vi "LINC Register LabVIEW File.vi"(4 "alternate packet names (empty)":string[](array[string]), 5 "ID":i32=-1, 6 "control names (empty)":string[](array[string]), 7 "mode (exclude)":enum16{"exclude", "include"}(ring), 8 "error in (no error)":errorcluster, 9 "type (CMD)":enum16{"CMD", "TLM", "CMD_HDR", "TLM_HDR"}(ring), 10 "prototype path":path, 11 "LINC session":refnum<class "LINC.lvclass">) -> (0 "error out":errorcluster, 3 "dup LINC session":refnum<class "LINC.lvclass">)   [LabVIEW 2018, in "STEPkgDriver_LINC.lvlib" / "LINC.lvclass"]
uses:
  LINC.lvclass
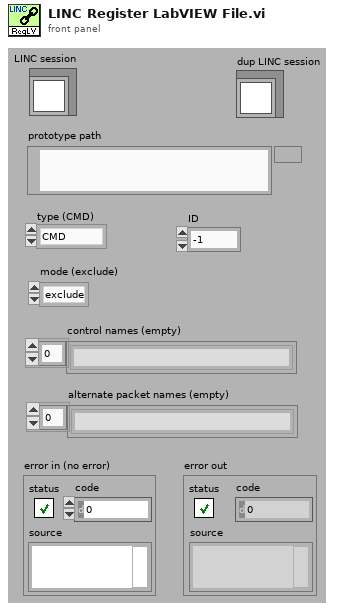
[diagram p1: front panel]
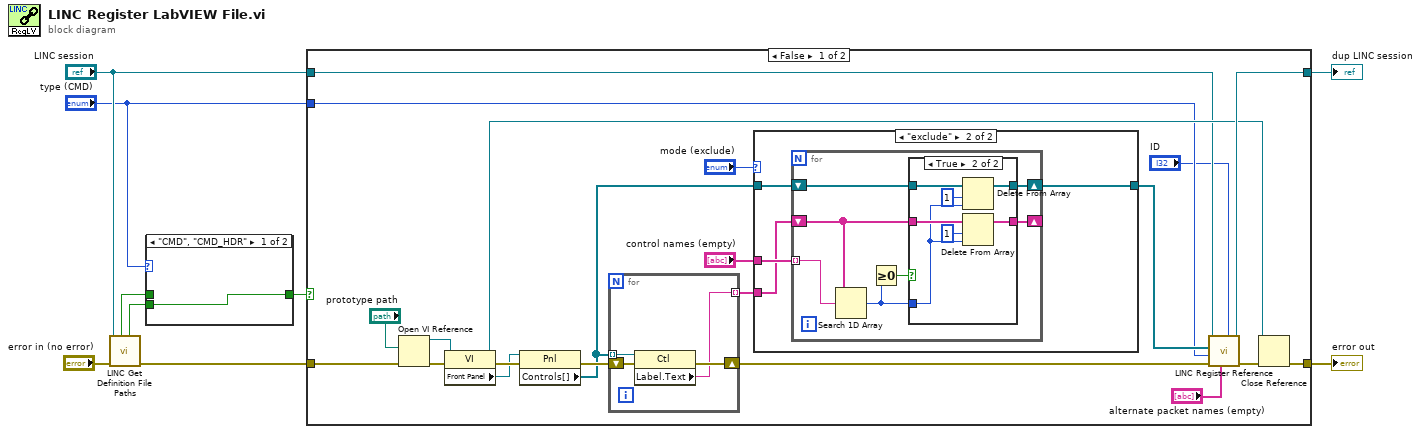
[diagram p0: block diagram]
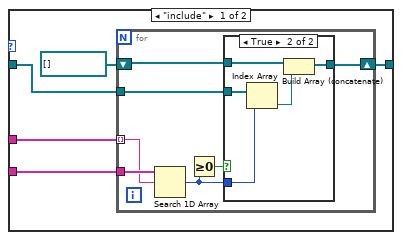
[diagram p2: hidden frame]
diagram:
  n1 = call "LINC Get Definition File Paths.vi"("error in (no error)"="error in (no error)", "LINC session"="LINC session") -> ("error out"=w5:errorcluster, "CMD definition exists"=w6:bool, "TLM definition exists"=w7:bool)  [unwired: 4 in, 3 out]
  n2 = case shown="\"CMD\", \"CMD_HDR\"" "type (CMD)" {
    tunnel: w7 -> [_ w11]
    tunnel: w6 -> [w10 _]
    tunnel: [w10 w11] -> w2
    frame "CMD", "CMD_HDR" {
    }
    frame "TLM", "TLM_HDR" {
    }
  }
  n3 = case shown="False" w2 {
    tunnel: [w20 w76] -> w9
    tunnel: [w19 w75] -> w8
    tunnel: w5 -> [w15 w76]
    tunnel: "LINC session" -> [w14 w75]
    tunnel: "type (CMD)" -> [w13 _]
    frame False {
      n4 = Open VI Reference(vi path="prototype path", error in (no error)=w15) -> (vi reference=w29:refnum<vi>, error out=w30:errorcluster)  [unwired: 1 in, 3 out]
      n5 = property class="VI"(reference=w29, error in=w30) -> (reference out=w17:refnum<vi>, error out=w32:errorcluster, "Front Panel"=w31:refnum<vi>)
      n6 = property class="Pnl"(reference=w31, error in=w32) -> (error out=w27:errorcluster, "Controls[]"=w24:refnum<vi>[])  [unwired: 1 out]
      n7 = for {
        shift-right: [w73] -> w22
        shift-left: w27 -> [w74]
        tunnel: w24 -> [w72] mode=indexing
        tunnel: [w71] -> w25 mode=indexing
        n8 = property class="Ctl"(reference=w72, error in=w74) -> (error out=w73:errorcluster, "Label.Text"=w71:string)  [unwired: 1 out]
      }
      n9 = case shown="\"exclude\"" "mode (exclude)" {
        tunnel: w25 -> [w36 w51]
        tunnel: w24 -> [w35 w52]
        tunnel: [w33 w53] -> w18
        tunnel: "control names (empty)" -> [w37 w54]
        frame "include" {
          n10 = for {
            tunnel: w37 -> [w43] mode=indexing
            tunnel: w36 -> [w44]
            tunnel: w35 -> [w42]
            shift-right: [w41] -> w33
            shift-left: refnum<vi>[] [] -> [w40]
            n11 = Search 1D Array(1D array=w44, element=w43) -> (index of element=w39:i32)  [unwired: 1 out]
            n12 = Greater Or Equal To 0?(x=w39) -> (x >= 0?=w38:bool)
            n13 = case shown="True" w38 {
              tunnel: w42 -> [_ w50]
              tunnel: w39 -> [_ w49]
              tunnel: [w45 w47] -> w41
              tunnel: w40 -> [w45 w46]
              frame False {
              }
              frame True {
                n14 = Index Array(array=w50, index=w49) -> (element=w48:refnum<vi>)
                n15 = Build Array (concatenate)(w46, w48) -> (w47:refnum<vi>[])
              }
            }
          }
        }
        frame "exclude" {
          n16 = for {
            tunnel: w54 -> [w61] mode=indexing
            shift-right: [w60] -> w53
            shift-left: w52 -> [w59]
            shift-right: [w55] -> _
            shift-left: w51 -> [w56]
            n17 = Search 1D Array(1D array=w56, element=w61) -> (index of element=w58:i32)  [unwired: 1 out]
            n18 = Greater Or Equal To 0?(x=w58) -> (x >= 0?=w57:bool)
            n19 = case shown="True" w57 {
              tunnel: w58 -> [_ w64]
              tunnel: [w63 w69] -> w60
              tunnel: w59 -> [w63 w70]
              tunnel: w56 -> [w62 w66]
              tunnel: [w62 w65] -> w55
              frame False {
              }
              frame True {
                n20 = Delete From Array(array=w70, length=1, index=w64) -> (array with subset deleted=w69:refnum<vi>[])  [unwired: 1 out]
                n21 = Delete From Array(array=w66, length=1, index=w64) -> (array with subset deleted=w65:string[])  [unwired: 1 out]
              }
            }
          }
        }
      }
      n22 = call "LINC Register Reference.vi"("ID"="ID", "alternate packet names (empty)"="alternate packet names (empty)", "error in (no error)"=w22, "type (CMD)"=w13, "controls"=w18, "LINC session"=w14) -> ("error out"=w21:errorcluster, "dup LINC session"=w19:refnum<class "LINC.lvclass">)  [unwired: 4 in]
      n23 = Close Reference(reference=w17, error in (no error)=w21) -> (error out=w20:errorcluster)
    }
    frame True {
    }
  }
  "error out" <- w9
  "dup LINC session" <- w8
